vi "Temp & pO2 Measurements.vi"() -> ()   [LabVIEW 2013]
doc: "This example configures the instrument to take one reading from its available parameter."
uses:
  Instance           7 31Saved   Temp & pO2 Measurements .vi
  Program Files/National Instruments/LabVIEW 2018/instr.lib/Keithley 2000/Keithley 2000.lvlib
  <vilib>/Utility/file.llb/Write Delimited Spreadsheet (DBL).vi
  Program Files/National Instruments/LabVIEW 2018/instr.lib/Keithley 2000/Public/Configure/Configure Route Single.vi
panel:
  in  "stop":bool
  out "Percent Complete":dbl=84.58333333333333 format="%_3f"
  in  "Length of Run (hh:mm)":dbl=3600.0 step=900.0 format="%<%H:%M>t"
  in  "Timmer On?":bool
  in  "Unit Address (1)":u8=1
  in  "VISA Resource: Eurotherm":refnum<visa-resource-name>="COM1"
  out "Sample Temp (C)":sgl=21.304764 format="%.3g"
  out "Sample Temp":sgl(graph)=21.304764
  in  "?":refnum<visa-resource-name>="GPIB0::14::INSTR"
  in  "O2 EMF Channel":i32=3
  out "Sensor EMF":dbl=0.00366675431 caption="O2 Sensor  EMF"
  out "Sensor Po2":dbl=-0.6089004780970528 caption="LogPO2 pressure"
  out "Sensor Po2 2":dbl(graph)=-0.6089004780970528
  in  "Measurement Peroid":dbl=3.0 caption="Delay Time (s)" format="%#_3f"
  in  "String":string
  out "Scan Number":i32=9
  # "seconds"
  # "File Comments:"
  # "Keithley 2000 Parameters"
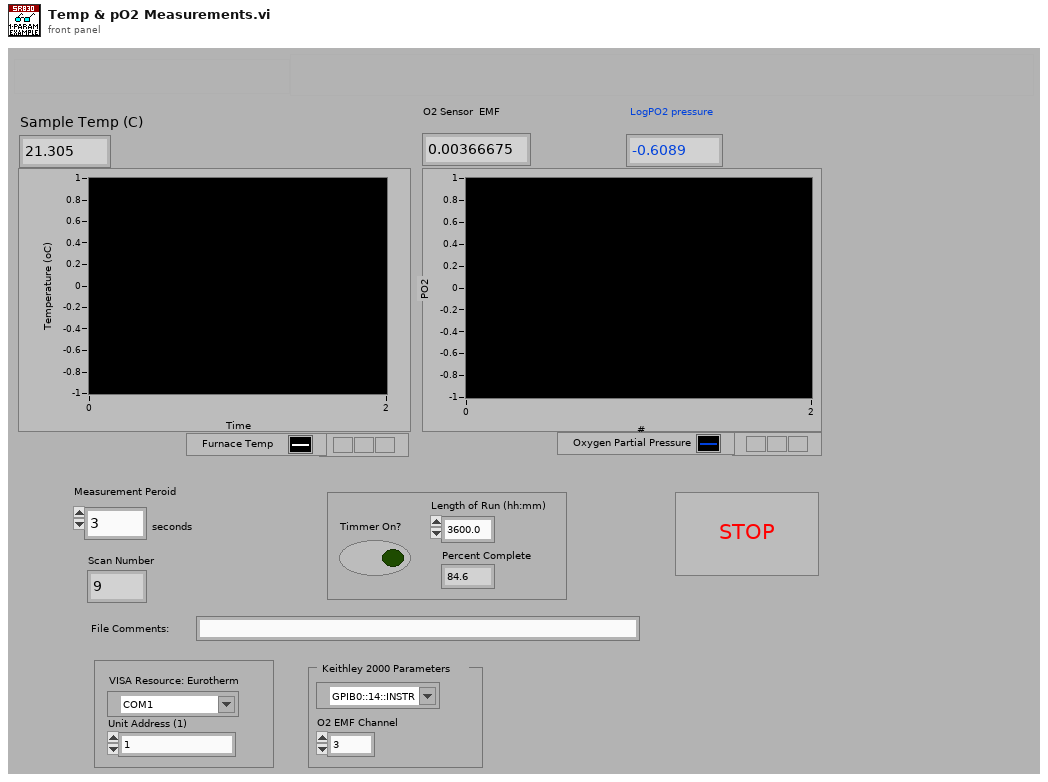
[diagram p1: front panel]
types:
  T1 = cluster{"Baud Rate (9600)":u32, "Parity (0: None)":u16, "Break Length (0)":u16}
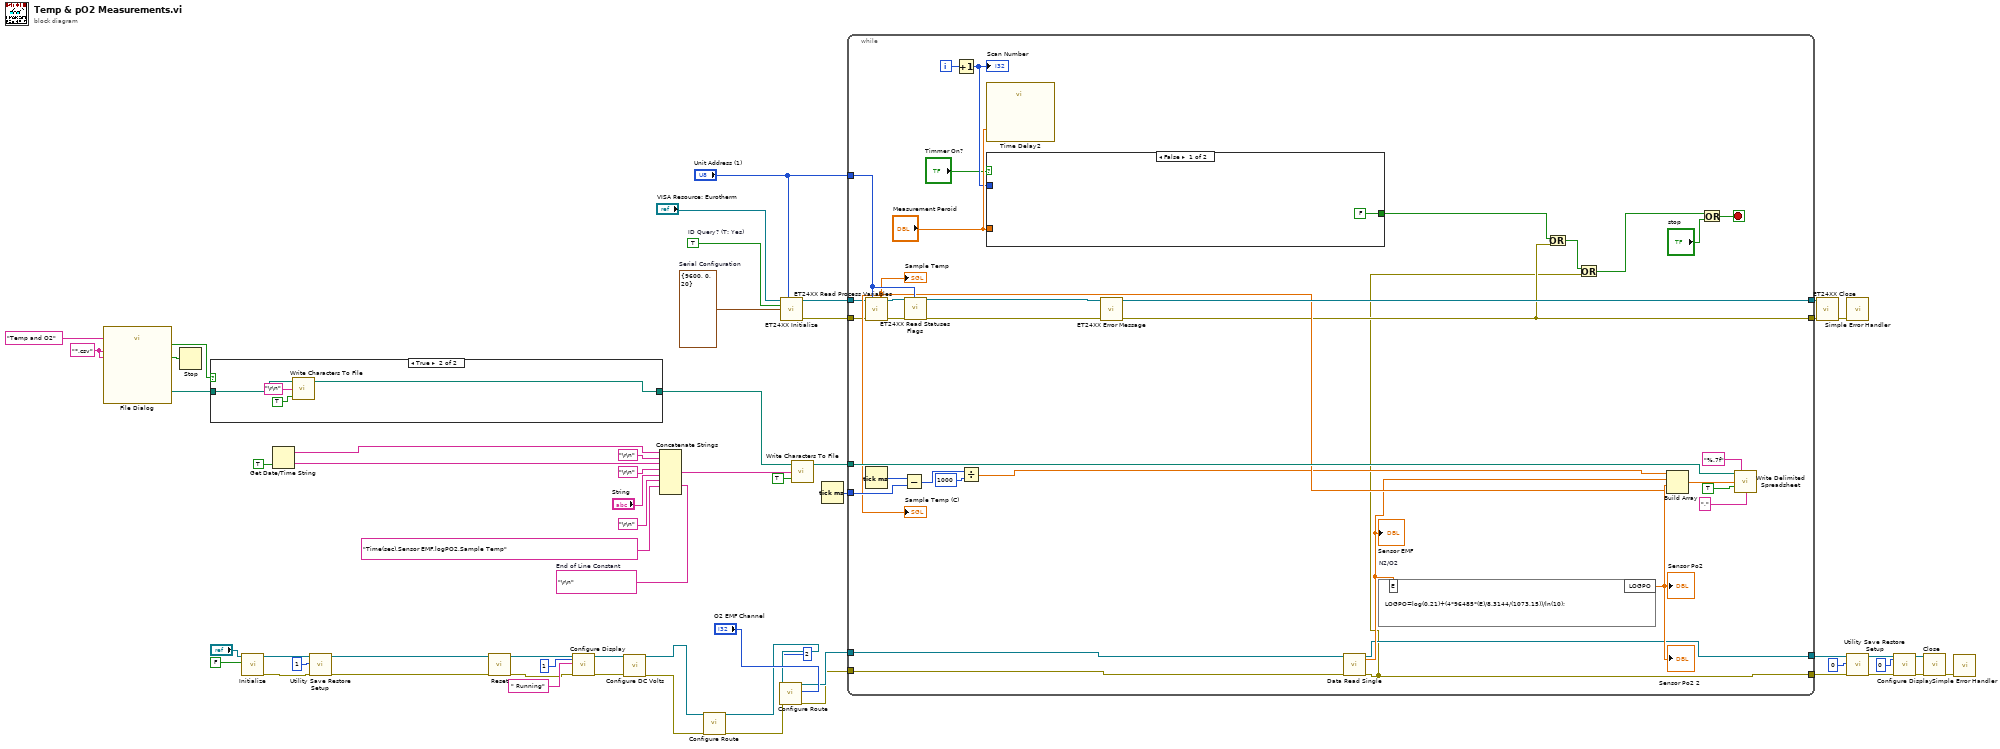
[diagram p0: block diagram]
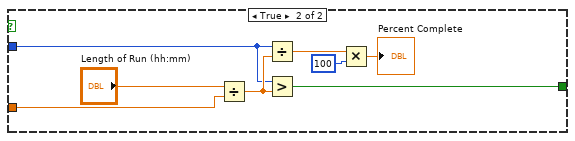
[diagram p3: hidden frame]
diagram:
  w23 = "*.csv"
  w46 = T1 {"Baud Rate (9600)"=9600, "Parity (0: None)"=0, "Break Length (0)"=20}  # Serial Configuration
  w48 = TRUE  # ID Query? (T: Yes)
  w53 = "\r\n"  # End of Line Constant
  n1 = call "File Dialog"("default name"="Temp and O2", "pattern (all files)"=w23, "pattern label"=w23) -> ("selected path"=w19:path, "exists"=w20:bool, "cancelled"=w21:bool)  [unwired: 9 in, 1 out]
  n2 = Stop(stop? (T)=w21) -> ()
  n3 = case shown="True" w20 {
    tunnel: w19 -> [w59 w61]
    tunnel: [w59 w60] -> w18
    frame False {
    }
    frame True {
      n4 = call <vilib>:"Write Characters To File.vi"("append to file? (new file:F)"=TRUE, "character string"="\r\n", "file path (dialog if empty)"=w61) -> ("new file path (Not A Path if cancelled)"=w60:path)  [unwired: 2 in]
    }
  }
  n5 = call "Initialize.vi"("VISA resource name"="?", "Reset? (T: Reset)"=FALSE) -> ("VISA resource name out"=w37:refnum<visa-resource-name>, "error out"=w13:errorcluster)  [unwired: 16 in]
  n6 = Get Date/Time String(want seconds? (F)=TRUE) -> (date string=w16:string, time string=w15:string)  [unwired: 2 in]
  n7 = call "Utility Save Restore Setup.vi"("VISA resource name"=w37, "Operation (0: Restore)"=1, "error in (no error)"=w13) -> ("VISA resource name out"=w14:refnum<visa-resource-name>, "error out"=w12:errorcluster)  [unwired: 15 in]
  n8 = call "Reset.vi"("VISA resource name"=w14, "error in (no error)"=w12) -> ("VISA resource name out"=w32:refnum<visa-resource-name>, "error out"=w11:errorcluster)  [unwired: 16 in]
  n9 = call "Configure Display.vi"("VISA resource name"=w32, "Display (0: Normal)"=1, "Text (empty)"=" Running", "error in (no error)"=w11) -> ("VISA resource name out"=w10:refnum<visa-resource-name>, "error out"=w9:errorcluster)  [unwired: 14 in]
  n10 = call "Configure DC Volts.vi"("VISA resource name"=w10, "error in (no error)"=w9) -> ("VISA resource name out"=w8:refnum<visa-resource-name>, "error out"=w7:errorcluster)  [unwired: 16 in]
  n11 = Concatenate Strings "Concatenate Strings"(w16, "\r\n", w15, "\r\n", "String", "\r\n", "Time(sec),Sensor EMF,logPO2,Sample Temp" ("string"), w53) -> (w57:string)
  n12 = call-poly "Configure Route.vi"("VISA resource name"=w8, "error in (no error)"=w7) -> ("VISA resource name out"=w5:refnum<visa-resource-name>, "error out"=w3:errorcluster)  [unwired: 16 in]
  n13 = call-poly "Configure Route.vi"("VISA resource name"=w5, "Operation (0: Open All)"=2 ("CH_Sensor_EMF 2"), "Channel (1)"="O2 EMF Channel", "error in (no error)"=w3) -> ("VISA resource name out"=w2:refnum<visa-resource-name>, "error out"=w1:errorcluster)  [unwired: 14 in]
  n14 = call "ET24XX Initialize.vi"("VISA resource name"="VISA Resource: Eurotherm", "Unit Address (1)"="Unit Address (1)", "ID Query? (T: Yes)"=w48, "Serial Configuration"=w46) -> ("VISA resource name out"=w44:refnum<visa-resource-name>, "error out"=w43:errorcluster)  [unwired: 10 in]
  n15 = call <vilib>:"Write Characters To File.vi"("append to file? (new file:F)"=TRUE, "character string"=w57, "file path (dialog if empty)"=w18) -> ("new file path (Not A Path if cancelled)"=w49:path)  [unwired: 2 in]
  n16 = Tick Count (ms)() -> (millisecond timer value=w58:u32)
  n17 = while {
    tunnel: w58 -> [w95]
    tunnel: w49 -> [w90]
    tunnel: [w67] -> w35
    tunnel: [w66] -> w34
    tunnel: "Unit Address (1)" -> [w85]
    tunnel: w44 -> [w81]
    tunnel: w43 -> [w80]
    tunnel: [w71] -> w42
    tunnel: [w84] -> w41
    tunnel: w2 -> [w65]
    tunnel: w1 -> [w64]
    i -> [w98]
    stop <- w77 stop-if-true
    n18 = call "ET24XX Read Process Variables.vi"("VISA resource name"=w81, "Unit Address (1)"=w85, "error in (no error)"=w80) -> ("Process Value"=w82:sgl, "VISA resource name out"=w86:refnum<visa-resource-name>, "error out"=w87:errorcluster)  [unwired: 6 in, 4 out]
    "Sample Temp (C)" <- w82
    "Sample Temp" <- w82
    n19 = Tick Count (ms)() -> (millisecond timer value=w97:u32)
    n20 = Subtract(x=w97, y=w95) -> (x-y=w96:u32)
    n21 = call "ET24XX Read Statuses Flags.vi"("VISA resource name"=w86, "error in (no error)"=w87, "Unit Address (1)"=w85) -> ("VISA resource name out"=w88:refnum<visa-resource-name>, "error out"=w89:errorcluster)  [unwired: 7 in, 8 out]
    n22 = Increment(x=w98) -> (x+1=w78:i32)
    "Scan Number" <- w78
    n23 = Divide(x=w96, y=u32 1000) -> (x/y=w68:dbl)
    n24 = call "Time Delay2"("Delay Time (s)"="Measurement Peroid") -> ()  [unwired: 10 in, 1 out]
    n25 = case shown="False" "Timmer On?" {
      tunnel: "Measurement Peroid" -> [_ w106]
      tunnel: w78 -> [_ w103]
      tunnel: [FALSE w105] -> w72
      frame False {
      }
      frame True {
        n26 = Divide(x="Length of Run (hh:mm)", y=w106) -> (x/y=w104:dbl)
        n27 = Divide(x=w103, y=w104) -> (x/y=w101:dbl)
        n28 = Greater?(x=w103, y=w104) -> (0:w105:bool)
        n29 = Multiply(x=w101, y=100) -> (x*y=→"Percent Complete":dbl)
      }
    }
    n30 = call "ET24XX Error Message.vi"("VISA session"=w88, "error in (no error)"=w89) -> ("dup VISA session"=w84:refnum<visa-resource-name>, "error out"=w71:errorcluster)  [unwired: 9 in, 3 out]
    n31 = call "Data Read Single.vi"("VISA resource name"=w65, "error in (no error)"=w64) -> ("VISA resource name out"=w67:refnum<visa-resource-name>, "Measurement"=w73:dbl, "error out"=w66:errorcluster)  [unwired: 13 in, 2 out]
    "Sensor EMF" <- w73
    n32 = formula code="LOGPO=log(0.21)+(4*96485*(E)/8.3144/(1073.15))/ln(10);" "N2/O2"("E"=w73) -> ("LOGPO"=w83:dbl)
    "Sensor Po2 2" <- w83
    "Sensor Po2" <- w83
    n33 = Or(x=w72, y=w71) -> (x .or. y?=w70:bool)
    n34 = Or(x=w70, y=w66) -> (x .or. y?=w69:bool)
    n35 = Build Array(w68, w73, w83, w82) -> (w91:dbl[])
    n36 = Or(x=w69, y="stop") -> (x .or. y?=w77:bool)
    n37 = call-poly <vilib>:"Write Delimited Spreadsheet.vi"("file path (dialog if empty)"=w90, "format (%.3f)"="%.7f", "1D data"=w91, "append to file? (new file:F)"=TRUE, "delimiter (\\t)"=",") -> ()  [unwired: 9 in, 2 out]
  }
  n38 = call "ET24XX Close.vi"("VISA resource name"=w41, "error in (no error)"=w42) -> ("error out"=w39:errorcluster)  [unwired: 13 in]
  n39 = call <vilib>:"Simple Error Handler.vi"("error in (no error)"=w39) -> ()  [unwired: 4 in, 5 out]
  n40 = call "Utility Save Restore Setup.vi"("VISA resource name"=w35, "Operation (0: Restore)"=0, "error in (no error)"=w34) -> ("VISA resource name out"=w26:refnum<visa-resource-name>, "error out"=w25:errorcluster)  [unwired: 15 in]
  n41 = call "Configure Display.vi"("VISA resource name"=w26, "Display (0: Normal)"=0, "error in (no error)"=w25) -> ("VISA resource name out"=w28:refnum<visa-resource-name>, "error out"=w27:errorcluster)  [unwired: 15 in]
  n42 = call "Close.vi"("VISA resource name"=w28, "error in (no error)"=w27) -> ("error out"=w40:errorcluster)  [unwired: 17 in]
  n43 = call <vilib>:"Simple Error Handler.vi"("error in (no error)"=w40) -> ()  [unwired: 4 in, 5 out]
